vi "Opgaven 6.vi"() -> ()   [LabVIEW 2023]
panel:
  in  "Unit to write":string
  in  "Path":path
  in  "String to write":string
  in  "Numeric to Wire":dbl
  out "Combined string":string
  out "Offset past match":i32
  out "Number out":dbl
  in  "String 2":string
  in  "Trailer":string
  in  "Header":string
  out "String lenght 4":i32
  in  "Numeric":dbl
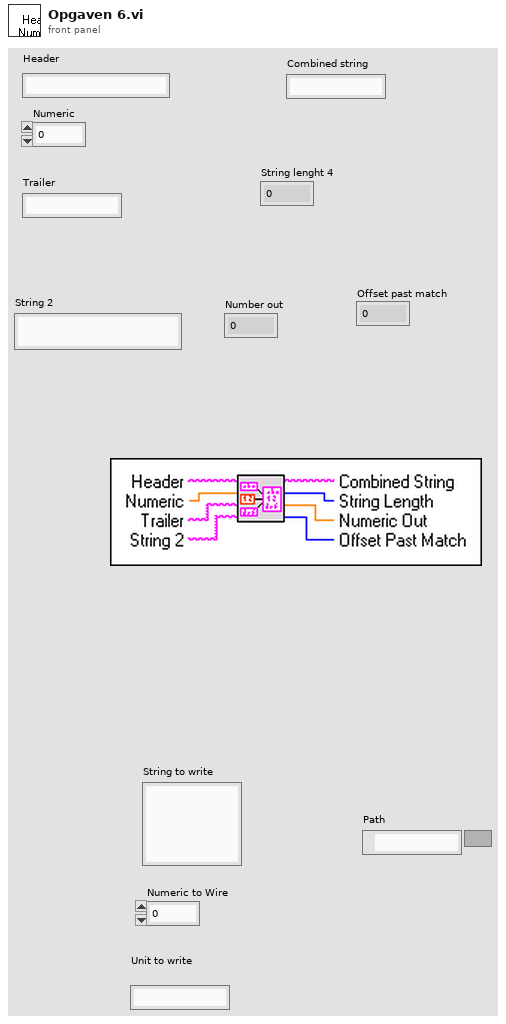
[diagram p1: front panel]
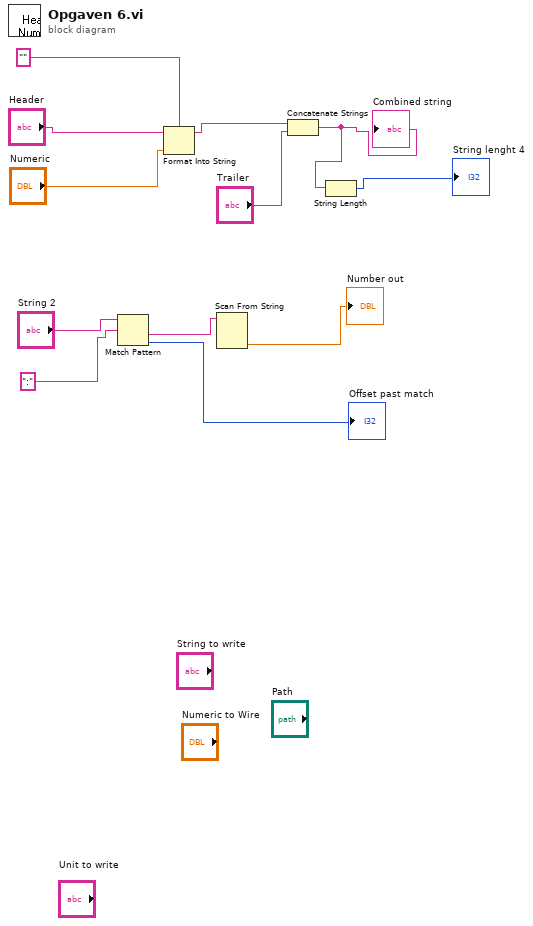
[diagram p0: block diagram]
diagram:
  n1 = Match Pattern(string="String 2", regular expression=":") -> (after substring=w5:string, offset past match=→"Offset past match":i32)  [unwired: 1 in, 2 out]
  n2 = Format Into String(format string="", initial string="Header", "Numeric") -> (resulting string=w10:string)  [unwired: 1 in, 1 out]
  n3 = Scan From String(input string=w5) -> (output 1=→"Number out":dbl)  [unwired: 4 in, 3 out]
  n4 = Concatenate Strings(w10, "Trailer") -> (w8:string)
  "Combined string" <- w8
  n5 = String Length(string=w8) -> (length=→"String lenght 4":i32)
